vi "PathPlanner_DriveFeedFwds_Interpolate.vi"(9 "Time":dbl, 10 "end Val":T1, 11 "in DriveFeedFwds":T1) -> (3 "interpolated DriveFeedFwds":T1)   [LabVIEW 2019, in "PathPlanner24.lvlib"]
doc: "Interpolate between this state and the given state\n \nInputs: \n - trajectoryState - cluster - this trajectory state\n - endVal - cluster - State to interpolate with\n - t - double - Interpolation factor (0.0-1.0)\n\nOutputs:\n - Interpolated state - trajectory state - interpolated state"
uses:
  PathPlanner24.lvlib
  TypeDef/PathPlannerDriveFeedFwds.ctl
  <vilib>/Rock Robotics/WPI/ThirdParty/JAS_Junk/TrajLib/Trajectory_Library.lvlib
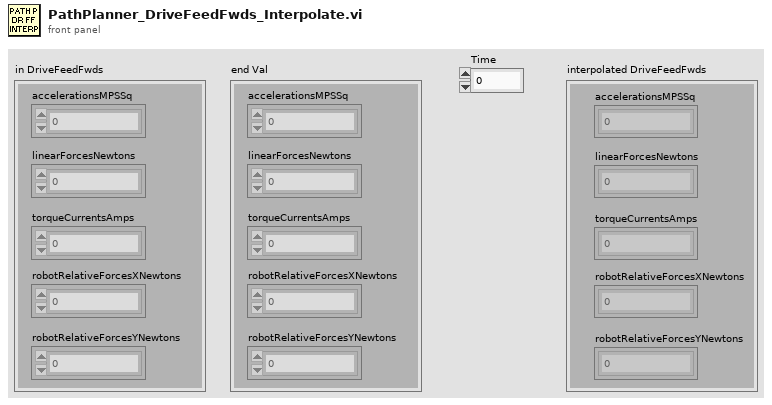
[diagram p1: front panel]
types:
  T1 = typedef "PathPlanner24.lvlib/PathPlannerDriveFeedFwds.ctl" = cluster{"accelerationsMPSSq":dbl[], "linearForcesNewtons":dbl[], "torqueCurrentsAmps":dbl[], "robotRelativeForcesXNewtons":dbl[], "robotRelativeForcesYNewtons":dbl[]}
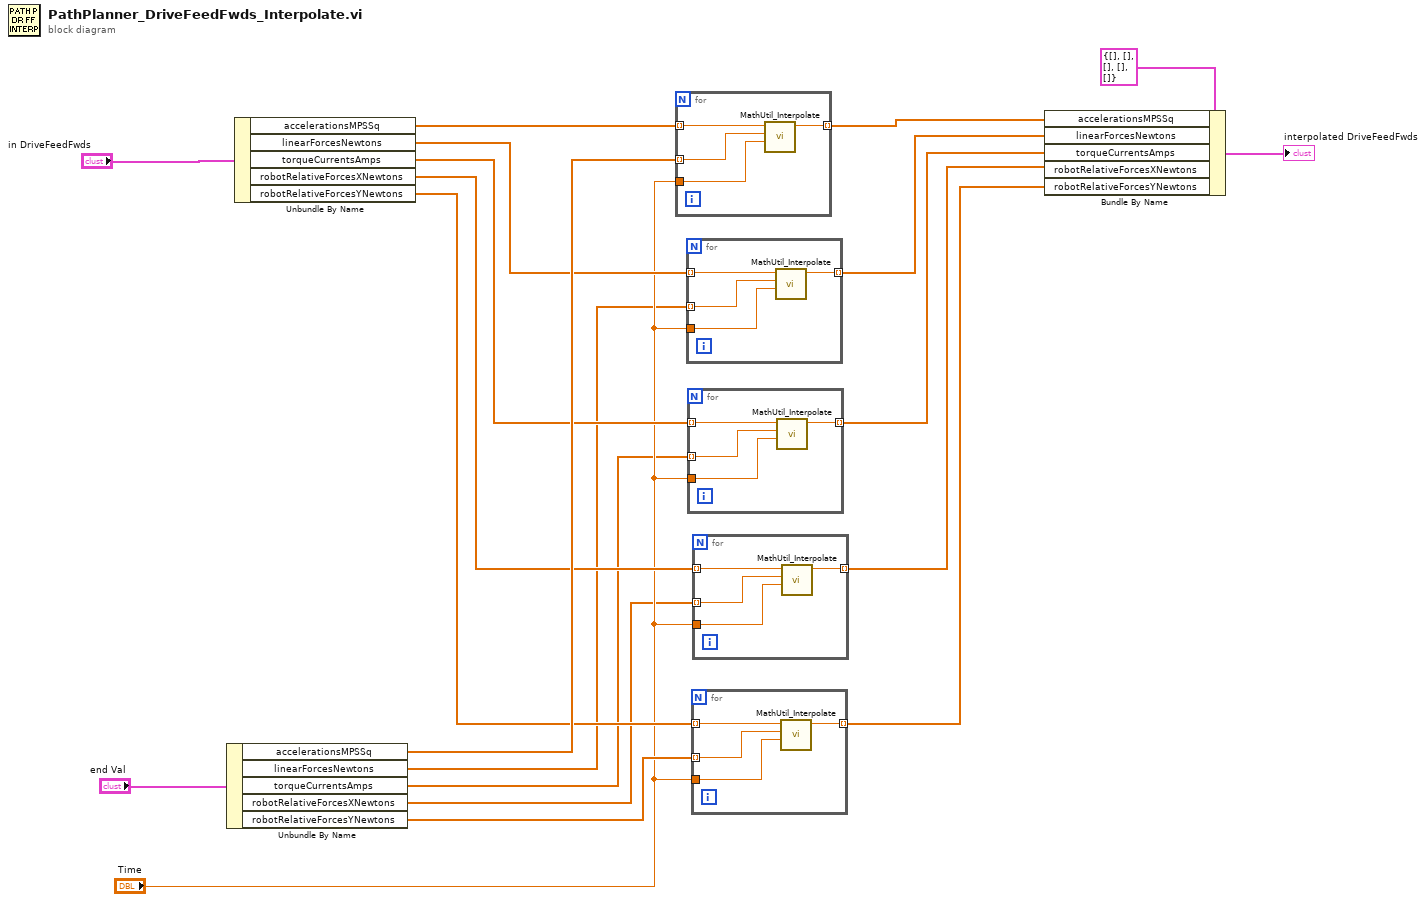
[diagram p0: block diagram]
diagram:
  n1 = Unbundle By Name("end Val") -> ("accelerationsMPSSq"=w16:dbl[], "linearForcesNewtons"=w7:dbl[], "torqueCurrentsAmps"=w8:dbl[], "robotRelativeForcesXNewtons"=w9:dbl[], "robotRelativeForcesYNewtons"=w11:dbl[])
  n2 = Unbundle By Name("in DriveFeedFwds") -> ("accelerationsMPSSq"=w17:dbl[], "linearForcesNewtons"=w15:dbl[], "torqueCurrentsAmps"=w14:dbl[], "robotRelativeForcesXNewtons"=w13:dbl[], "robotRelativeForcesYNewtons"=w12:dbl[])
  n3 = for {
    tunnel: w17 -> [w24] mode=indexing
    tunnel: w16 -> [w23] mode=indexing
    tunnel: "Time" -> [w22]
    tunnel: [w21] -> w6 mode=indexing
    n4 = call <vilib>:"MathUtil_Interpolate.vi"("T"=w22, "EndValue"=w23, "StartValue"=w24) -> ("InterpolatedValue"=w21:dbl)  [unwired: 8 in]
  }
  n5 = for {
    tunnel: w15 -> [w28] mode=indexing
    tunnel: w7 -> [w27] mode=indexing
    tunnel: "Time" -> [w26]
    tunnel: [w25] -> w5 mode=indexing
    n6 = call <vilib>:"MathUtil_Interpolate.vi"("T"=w26, "EndValue"=w27, "StartValue"=w28) -> ("InterpolatedValue"=w25:dbl)  [unwired: 8 in]
  }
  n7 = for {
    tunnel: w14 -> [w32] mode=indexing
    tunnel: w8 -> [w31] mode=indexing
    tunnel: "Time" -> [w30]
    tunnel: [w29] -> w4 mode=indexing
    n8 = call <vilib>:"MathUtil_Interpolate.vi"("T"=w30, "EndValue"=w31, "StartValue"=w32) -> ("InterpolatedValue"=w29:dbl)  [unwired: 8 in]
  }
  n9 = for {
    tunnel: w12 -> [w36] mode=indexing
    tunnel: w11 -> [w35] mode=indexing
    tunnel: "Time" -> [w34]
    tunnel: [w33] -> w2 mode=indexing
    n10 = call <vilib>:"MathUtil_Interpolate.vi"("T"=w34, "EndValue"=w35, "StartValue"=w36) -> ("InterpolatedValue"=w33:dbl)  [unwired: 8 in]
  }
  n11 = for {
    tunnel: w13 -> [w40] mode=indexing
    tunnel: w9 -> [w39] mode=indexing
    tunnel: "Time" -> [w38]
    tunnel: [w37] -> w3 mode=indexing
    n12 = call <vilib>:"MathUtil_Interpolate.vi"("T"=w38, "EndValue"=w39, "StartValue"=w40) -> ("InterpolatedValue"=w37:dbl)  [unwired: 8 in]
  }
  n13 = Bundle By Name(cluster=T1 {"accelerationsMPSSq"=[], "linearForcesNewtons"=[], "torqueCurrentsAmps"=[], "robotRelativeForcesXNewtons"=[], "robotRelativeForcesYNewtons"=[]} ("PathPlannerState"), "accelerationsMPSSq"=w6, "linearForcesNewtons"=w5, "torqueCurrentsAmps"=w4, "robotRelativeForcesXNewtons"=w3, "robotRelativeForcesYNewtons"=w2) -> (→"interpolated DriveFeedFwds":T1)
